vi "Demo.vi"() -> ()   [LabVIEW 2020, in "Tree Helpers.lvlib" / "File Tree.lvclass"]
uses:
  File Tree.lvclass
  File Tree.lvclass/File Tree.ctl
panel:
  in  "absolute?":bool
  out "Selected Tags":string[](array[string])
  in  "Tree":string[](tree)
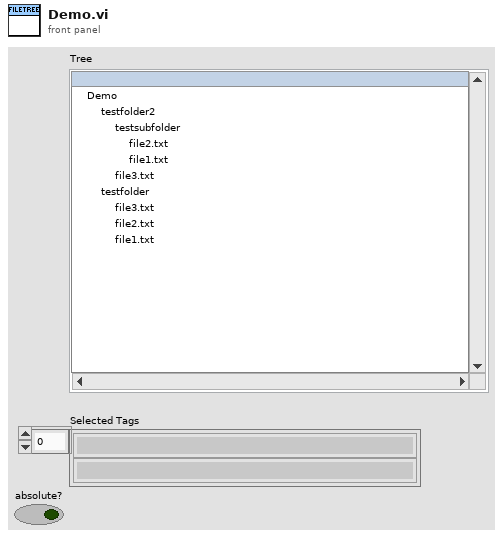
[diagram p1: front panel]
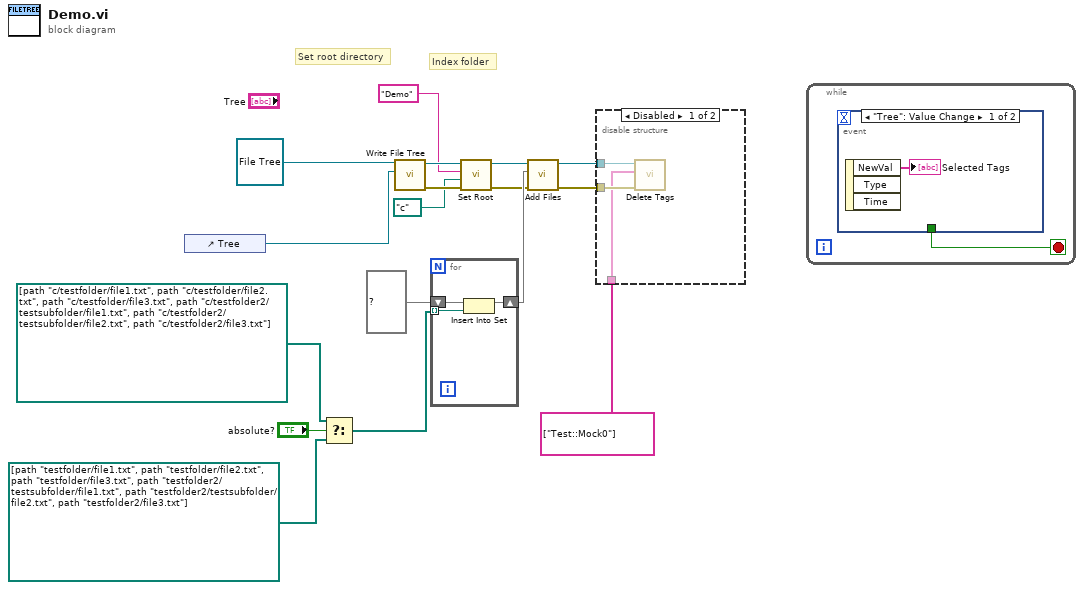
[diagram p0: block diagram]
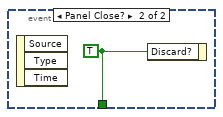
[diagram p2: hidden frame]
diagram:
  # "Set root directory"
  # "Index folder"
  n1 = control-ref of="Tree"() -> (w16:refnum<vi>)
  n2 = Select(t=path[] [path "c:/testfolder/file1.txt", path "c:/testfolder/file2.txt", path "c:/testfolder/file3.txt", path "c:/testfolder2/testsubfolder/file1.txt", path "c:/testfolder2/testsubfolder/file2.txt", path "c:/testfolder2/file3.txt"], s="absolute?", f=path[] [path "testfolder/file1.txt", path "testfolder/file2.txt", path "testfolder/file3.txt", path "testfolder2/testsubfolder/file1.txt", path "testfolder2/testsubfolder/file2.txt", path "testfolder2/file3.txt"]) -> (s? t:f=w1:path[])
  n3 = call "Write File Tree.vi"("File Tree Reference"=w16, "File Tree In"=refnum<class "File Tree.lvclass"> refnum ("Support Utilities.lvlib:Tag Tree.lvclass")) -> ("error out"=w8:errorcluster, "File Tree Out"=w15:refnum<class "File Tree.lvclass">)  [unwired: 8 in]
  n4 = for {
    tunnel: w1 -> [w20] mode=indexing
    shift-right: [w18] -> w10
    shift-left: set{path} {} ("set in") -> [w19]
    n5 = Insert Into Set(10:w20, 11:w19) -> (3:w18:set{path})  [unwired: 1 out]
  }
  n6 = call "Set Root.vi"("error in (no error)"=w8, "Root Path"=path "c:/", "Root Name"="Demo", "File Tree In"=w15) -> ("error out"=w7:errorcluster, "File Tree Out"=w9:refnum<class "File Tree.lvclass">)  [unwired: 6 in]
  n7 = call "Add Files.vi"("error in (no error)"=w7, "Files"=w10, "File Tree In"=w9) -> ("error out"=w13:errorcluster, "File Tree Out"=w14:refnum<class "File Tree.lvclass">)  [unwired: 7 in]
  n8 = disable-structure "Diagram Disable Structure" shown="Disabled" {
    disable-tunnel: w14 -> [w23 _]
    disable-tunnel: w13 -> [w22 _]
    disable-tunnel: string[] ["Test::Mock0"] ("Tag") -> [w21 _]
    frame Disabled {
      n9 = call "Delete Tags.vi"("error in (no error)"=w22, "Tag"=w21, "File Tree In"=w23) -> ()  [unwired: 7 in, 2 out]
    }
    frame Enabled {
    }
  }
  n10 = while {
    stop <- w24 stop-if-true
    n11 = event shown="[0] \"Tree\": Value Change" {
      selector: _ -> [_ _]
      dyn-events: _ -> [_ _]
      timeout: _ -> [_ _]
      tunnel: [_ w26] -> w24
      event "Tree": Value Change {
        n12 = event-data() -> ("NewVal"=→"Selected Tags":string[])  [unwired: 1 in, 2 out]
      }
      event Panel Close? {
        w26 = TRUE ("Discard?")
        n13 = event-data() -> ()  [unwired: 1 in, 3 out]
        n14 = event-data ("Event Filter Node")("Discard?"=w26) -> ()  [unwired: 1 in, 1 out]
      }
    }
  }
